vi "氨氮报警信息.vi"(8 "error in (no error)":errorcluster, 11 "data in":T1) -> (0 "error out":errorcluster)   [LabVIEW 2016, in "斯坦道氨氮.lvlib"]
uses:
  <vilib>/Utility/sysdir.llb/System Directory Type.ctl
  <vilib>/addons/database/Auxilliary.llb/DB Tools Transaction.ctl
  <vilib>/addons/database/Auxilliary.llb/DB Tools Isolation Level.ctl
  <vilib>/addons/database/Auxilliary.llb/DB Tools Column Info.ctl
  <vilib>/addons/database/Auxilliary.llb/DB Tools DataTypes.ctl
  <vilib>/addons/database/Auxilliary.llb/DB Tools Parameter Info.ctl
  <vilib>/addons/database/Auxilliary.llb/DB Tools Parameter Dir.ctl
  <vilib>/addons/database/Connection.llb/DB Tools Open Connec (String).vi
  <vilib>/addons/database/Connection.llb/Conn Transaction.vi
  <vilib>/addons/database/Connection.llb/Conn Execute.vi
  <vilib>/addons/database/Recordset.llb/Rec Destroy - Connection.vi
  <vilib>/addons/database/Command.llb/Cmd Set Parameter Value (C).vi
  <vilib>/addons/database/Command.llb/Cmd Execute.vi
  <vilib>/addons/database/Recordset.llb/Rec Destroy - Command.vi
  <vilib>/addons/database/Command.llb/Cmd Delete.vi
  <vilib>/addons/database/Auxilliary.llb/DB Tools Format Datetime String (Time Stamp).vi
  <vilib>/addons/database/NI_Database_API.lvlib
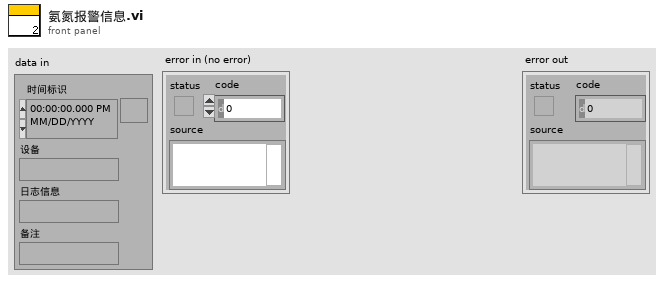
[diagram p1: front panel]
types:
  T1 = cluster{"时间标识":timestamp, "设备":string, "日志信息":string, "备注":string}
  T2 = typedef "NI_Database_API.lvlib/DB Tools Column Info.ctl" = cluster{"column name":string, "data type":T3, "size":i32, "allow null?":bool}
  T3 = typedef "NI_Database_API.lvlib/DB Tools DataTypes.ctl" = enum16{"String", "Long (I32)", "Single (SGL)", "Double (DBL)", "Date/Time", "Binary"}
  T4 = typedef "NI_Database_API.lvlib/DB Tools Isolation Level.ctl" = enum16{"chaos", "read uncommitted", "read committed", "repeatable read", "serializable"}
  T5 = typedef "NI_Database_API.lvlib/DB Tools Transaction.ctl" = enum16{"begin", "commit", "rollback"}
  T6 = typedef "System Directory Type.ctl" = i32
  T7 = typedef "NI_Database_API.lvlib/Conn ObjectReference.ctl" = refnum<k1>
  T8 = typedef "NI_Database_API.lvlib/DB Tools Parameter Info.ctl" = cluster{"parameter name":string, "type":T3, "direction":T9, "value":variant}
  T9 = typedef "NI_Database_API.lvlib/DB Tools Parameter Dir.ctl" = enum32{"Input", "Output", "Input/Output", "Return Value"}
  T10 = typedef "NI_Database_API.lvlib/Rec ObjectReference.ctl" = refnum<k1>
  T11 = typedef "NI_Database_API.lvlib/Cmd ObjectReference.ctl" = refnum<k1>
  T12 = typedef "NI_Database_API.lvlib/Cmd-Rec Object Reference.ctl" = refnum<k1>
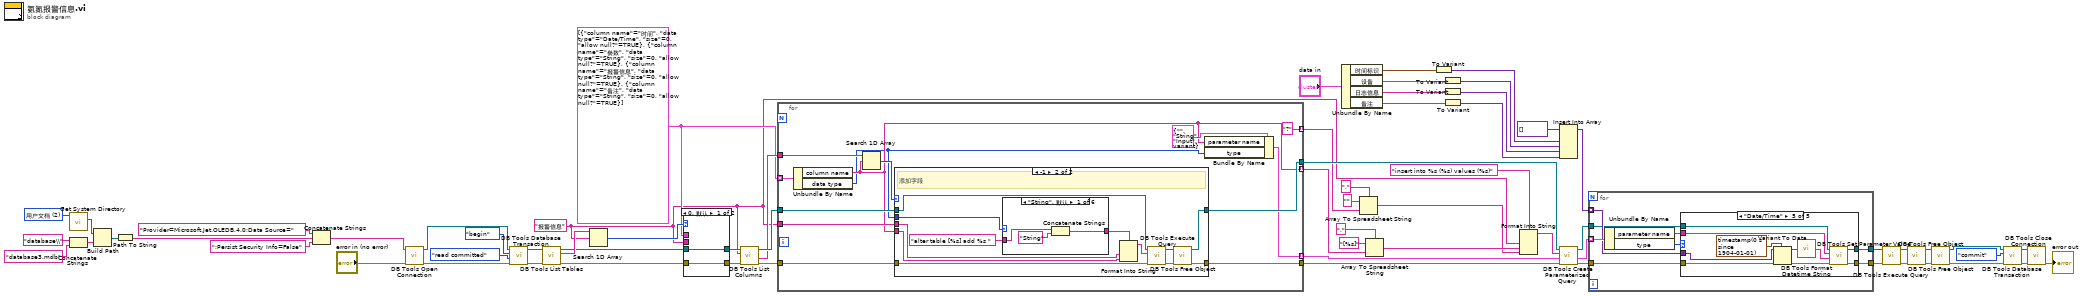
[diagram p0: block diagram]
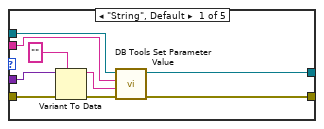
[diagram p2: hidden frame]
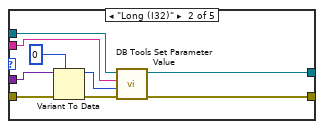
[diagram p3: hidden frame]
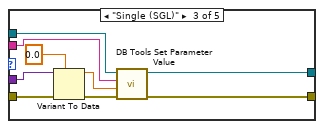
[diagram p4: hidden frame]
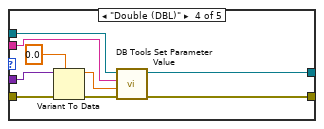
[diagram p5: hidden frame]
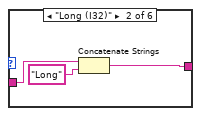
[diagram p7: hidden frame]
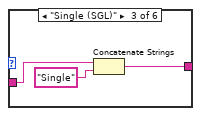
[diagram p8: hidden frame]
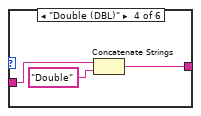
[diagram p9: hidden frame]
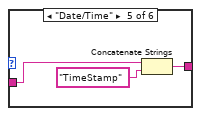
[diagram p10: hidden frame]
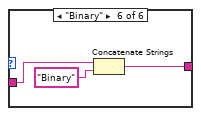
[diagram p11: hidden frame]
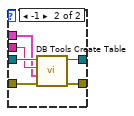
[diagram p12: hidden frame]
diagram:
  w44 = T2[] [{"column name"="时间", "data type"=enum."Date/Time", "size"=0, "allow null?"=TRUE}, {"column name"="参数", "data type"=enum."String", "size"=0, "allow null?"=TRUE}, {"column name"="报警信息", "data type"=enum."String", "size"=0, "allow null?"=TRUE}, {"column name"="备注", "data type"=enum."String", "size"=0, "allow null?"=TRUE}] ("column information")
  w37 = "报警信息"
  w66 = T6 2 items=["用户目录"=0, "用户桌面"=1, "用户文档"=2, "用户应用程序数据"=3, "用户设置"=4, "用户临时目录"=5, "公共文档"=6, "公共应用程序数据"=7, "公共设置"=8, "公共缓存"=13, "系统核心库"=9, "系统安装库"=10, "应用程序文件"=11, "启动盘根目录"=12] ("system directory type")
  n1 = call <vilib>:"Get System Directory.vi"("system directory type"=w66) -> ("system directory"=w64:path)  [unwired: 10 in]
  n2 = Concatenate Strings("database\\" ("condition"), "database3.mdb" ("database")) -> (w58:string)
  n3 = Build Path(base path=w64, name or relative path=w58) -> (appended path=w63:path)
  n4 = Path To String(path=w63) -> (string=w62:string)
  n5 = Concatenate Strings("Provider=Microsoft.Jet.OLEDB.4.0;Data Source=" ("condition"), w62, ";Persist Security Info=False" ("condition")) -> (w60:string)
  n6 = call-poly <vilib>:"DB Tools Open Connection.vi"("error in (no error)"="error in (no error)", "connection information"=w60) -> ("error out"=w2:errorcluster, "connection reference"=w4:T7)  [unwired: 6 in]
  n7 = call-poly <vilib>:"DB Tools Database Transaction.vi"("error in (no error)"=w2, "isolation level (chaos)"=DB_Tools_Isolation_Level."read committed", "operation (begin)"=DB_Tools_Transaction."begin", "connection reference"=w4) -> ("error out"=w1:errorcluster, "connection reference out"=w3:T7)  [unwired: 2 in]
  n8 = call <vilib>:"DB Tools List Tables.vi"("error in (no error)"=w1, "connection reference"=w3) -> ("error out"=w48:errorcluster, "tables"=w51:string[], "connection reference out"=w49:T7)  [unwired: 3 in]
  n9 = Search 1D Array(1D array=w51, element=w37) -> (index of element=w50:i32)  [unwired: 1 in]
  n10 = case shown="0, 默认" w50 {
    tunnel: w49 -> [w69 w75]
    tunnel: w48 -> [w68 w74]
    tunnel: w37 -> [_ w73]
    tunnel: w44 -> [_ w72]
    tunnel: [w69 w71] -> w43
    tunnel: [w68 w70] -> w42
    frame 0, Default {
    }
    frame -1 {
      n11 = call <vilib>:"DB Tools Create Table.vi"("error in (no error)"=w74, "column information"=w72, "table"=w73, "connection reference"=w75) -> ("error out"=w70:errorcluster, "connection reference out"=w71:T7)  [unwired: 4 in]
    }
  }
  n12 = call <vilib>:"DB Tools List Columns.vi"("error in (no error)"=w42, "table"=w37, "connection reference"=w43) -> ("error out"=w45:errorcluster, "columns"=w46:string[], "connection reference out"=w47:T7)  [unwired: 1 in, 1 out]
  n13 = for {
    tunnel: w47 -> [w86]
    tunnel: w46 -> [w88]
    tunnel: w45 -> [w85]
    tunnel: [w84] -> w41
    tunnel: [w83] -> w40
    tunnel: w37 -> [w82]
    tunnel: w44 -> [w81] mode=indexing
    tunnel: [w79] -> w39 mode=indexing
    tunnel: [w78] -> w32 mode=indexing
    tunnel: ["?"] -> w30 mode=indexing
    n14 = Unbundle By Name(w81) -> ("column name"=w78:string, "data type"=w76:T3)
    n15 = Search 1D Array(1D array=w88, element=w78) -> (index of element=w87:i32)  [unwired: 1 in]
    n16 = case shown="-1" w87 {
      tunnel: [w90 w99] -> w83
      tunnel: [w89 w98] -> w84
      tunnel: w86 -> [w90 w97]
      tunnel: w78 -> [_ w96]
      tunnel: w85 -> [w89 w95]
      tunnel: w82 -> [_ w94]
      tunnel: w76 -> [_ w92]
      frame 0, Default {
      }
      frame -1 {
        # "添加字段"
        n17 = case shown="\"String\", 默认" w92 {
          tunnel: "alter table [%s] add %s " -> [w105 w108 w111 w114 w117 w120]
          tunnel: [w104 w107 w110 w113 w116 w119] -> w91
          frame "String", Default {
            n18 = Concatenate Strings(w105, "String" ("字符串")) -> (w104:string)
          }
          frame "Long (I32)" {
            n19 = Concatenate Strings(w108, "Long" ("字符串")) -> (w107:string)
          }
          frame "Single (SGL)" {
            n20 = Concatenate Strings(w111, "Single" ("字符串")) -> (w110:string)
          }
          frame "Double (DBL)" {
            n21 = Concatenate Strings(w114, "Double" ("字符串")) -> (w113:string)
          }
          frame "Date/Time" {
            n22 = Concatenate Strings(w117, "TimeStamp" ("字符串")) -> (w116:string)
          }
          frame "Binary" {
            n23 = Concatenate Strings(w120, "Binary" ("字符串")) -> (w119:string)
          }
        }
        n24 = Format Into String(format string=w91, w94, w96) -> (resulting string=w100:string)  [unwired: 2 in, 1 out]
        n25 = call-poly <vilib>:"DB Tools Execute Query.vi"("error in (no error)"=w95, "SQL query"=w100, "connection reference"=w97) -> ("error out"=w101:errorcluster, "recordset reference"=w102:T10)  [unwired: 5 in]
        n26 = call-poly <vilib>:"DB Tools Free Object.vi"("error in (no error)"=w101, "recordset reference"=w102) -> ("error out"=w98:errorcluster, "connection reference"=w99:T7)  [unwired: 8 in]
      }
    }
    n27 = Bundle By Name(cluster=T8 {"parameter name"="", "type"=enum."String", "direction"=enum."Input", "value"=variant} ("parameter information"), "parameter name"=w78, "type"=w76) -> (w79:T8)
  }
  n28 = Unbundle By Name("data in") -> ("时间标识"=w24:timestamp, "设备"=w21:string, "日志信息"=w22:string, "备注"=w23:string)
  n29 = Array To Spreadsheet String(delimiter (Tab)="," ("分隔符(Tab)"), array=w30, 3:"" ("格式字符串")) -> (spreadsheet string=w29:string)
  n30 = Array To Spreadsheet String(delimiter (Tab)="," ("分隔符(Tab)"), array=w32, 3:"[%s]" ("格式字符串")) -> (spreadsheet string=w31:string)
  n31 = To Variant(anything=w24) -> (Variant=w19:variant)
  n32 = To Variant(anything=w21) -> (Variant=w18:variant)
  n33 = To Variant(anything=w22) -> (Variant=w17:variant)
  n34 = To Variant(anything=w23) -> (Variant=w16:variant)
  n35 = Format Into String(format string="insert into %s (%s) values (%s)" ("格式字符串"), w37, w31, w29) -> (resulting string=w28:string)  [unwired: 2 in, 1 out]
  n36 = Insert Into Array(array=variant[] [], new element #1=w19, new element #2=w18, new element #3=w17, new element #4=w16) -> (w15:variant[])  [unwired: 1 in]
  n37 = call <vilib>:"DB Tools Create Parameterized Query.vi"("error in (no error)"=w41, "parameters"=w39, "SQL query"=w28, "connection reference"=w40) -> ("error out"=w26:errorcluster, "parameters out"=w25:T8[], "command reference"=w27:T11)  [unwired: 3 in]
  n38 = for {
    tunnel: w27 -> [w125]
    tunnel: w26 -> [w123]
    tunnel: w25 -> [w128] mode=indexing
    tunnel: w15 -> [w126] mode=indexing
    tunnel: [w122] -> w14
    tunnel: [w121] -> w13
    n39 = Unbundle By Name(w128) -> ("parameter name"=w124:string, "type"=w127:T3)
    n40 = case shown="\"Date/Time\"" w127 {
      tunnel: w126 -> [w132 w140 w147 w157 w174]
      tunnel: w125 -> [w135 w144 w151 w161 w172]
      tunnel: w124 -> [w134 w143 w150 w156 w171]
      tunnel: w123 -> [w129 w138 w148 w158 w169]
      tunnel: [w131 w142 w152 w160 w168] -> w122
      tunnel: [w130 w141 w149 w159 w167] -> w121
      frame "String", Default {
        n41 = Variant To Data(error in=w129, type="", Variant=w132) -> (data=w133:string, error out=w137:errorcluster)
        n42 = call-poly <vilib>:"DB Tools Set Parameter Value.vi"("error in (no error)"=w137, "value"=w133, "parameter index"=w134, "command reference"=w135) -> ("error out"=w130:errorcluster, "command reference out"=w131:T11)  [unwired: 4 in]
      }
      frame "Long (I32)" {
        n43 = Variant To Data(error in=w138, type=0, Variant=w140) -> (data=w145:i32, error out=w146:errorcluster)
        n44 = call-poly <vilib>:"DB Tools Set Parameter Value.vi"("error in (no error)"=w146, "value"=w145, "parameter index"=w143, "command reference"=w144) -> ("error out"=w141:errorcluster, "command reference out"=w142:T11)  [unwired: 4 in]
      }
      frame "Single (SGL)" {
        n45 = Variant To Data(error in=w148, type=sgl 0.0, Variant=w147) -> (data=w154:sgl, error out=w155:errorcluster)
        n46 = call-poly <vilib>:"DB Tools Set Parameter Value.vi"("error in (no error)"=w155, "value"=w154, "parameter index"=w150, "command reference"=w151) -> ("error out"=w149:errorcluster, "command reference out"=w152:T11)  [unwired: 4 in]
      }
      frame "Double (DBL)" {
        n47 = Variant To Data(error in=w158, type=0.0, Variant=w157) -> (data=w163:dbl, error out=w164:errorcluster)
        n48 = call-poly <vilib>:"DB Tools Set Parameter Value.vi"("error in (no error)"=w164, "value"=w163, "parameter index"=w156, "command reference"=w161) -> ("error out"=w159:errorcluster, "command reference out"=w160:T11)  [unwired: 4 in]
      }
      frame "Date/Time" {
        n49 = Variant To Data(error in=w169, type=timestamp(0 s since 1904-01-01) ("时间标识"), Variant=w174) -> (data=w166:timestamp, error out=w170:errorcluster)
        n50 = call-poly <vilib>:"DB Tools Format Datetime String.vi"("time stamp"=w166) -> ("date/time string"=w165:string)
        n51 = call-poly <vilib>:"DB Tools Set Parameter Value.vi"("error in (no error)"=w170, "value"=w165, "parameter index"=w171, "command reference"=w172) -> ("error out"=w167:errorcluster, "command reference out"=w168:T11)  [unwired: 4 in]
      }
    }
  }
  n52 = call-poly <vilib>:"DB Tools Execute Query.vi"("error in (no error)"=w13, "command reference"=w14) -> ("error out"=w11:errorcluster, "command-recordset reference"=w12:T12)  [unwired: 6 in]
  n53 = call-poly <vilib>:"DB Tools Free Object.vi"("error in (no error)"=w11, "command-recordset reference"=w12) -> ("error out"=w9:errorcluster, "command reference"=w10:T11)  [unwired: 8 in]
  n54 = call-poly <vilib>:"DB Tools Free Object.vi"("error in (no error)"=w9, "command reference"=w10) -> ("error out"=w5:errorcluster, "connection reference"=w6:T7)  [unwired: 8 in]
  n55 = call-poly <vilib>:"DB Tools Database Transaction.vi"("error in (no error)"=w5, "operation (begin)"=DB_Tools_Transaction."commit", "connection reference"=w6) -> ("error out"=w7:errorcluster, "connection reference out"=w8:T7)  [unwired: 3 in]
  n56 = call <vilib>:"DB Tools Close Connection.vi"("error in (no error)"=w7, "connection reference"=w8) -> ("error out"=→"error out":errorcluster)  [unwired: 5 in]
